vi "test Init 1.vi"(11 "Test Case In":refnum<class "test Init.lvclass">) -> (0 "error out":errorcluster, 3 "Test Case Out":refnum<class "test Init.lvclass">)   [LabVIEW 2023, in "test Init.lvclass"]
uses:
  test Init.lvclass
  test Init.lvclass/test Init.ctl
  <vilib>/Astemes/LUnit/Test Case.lvclass
  source/Base Graph/Base Graph.lvclass
panel:
  out "Intensity Graph":dbl[][](graph)
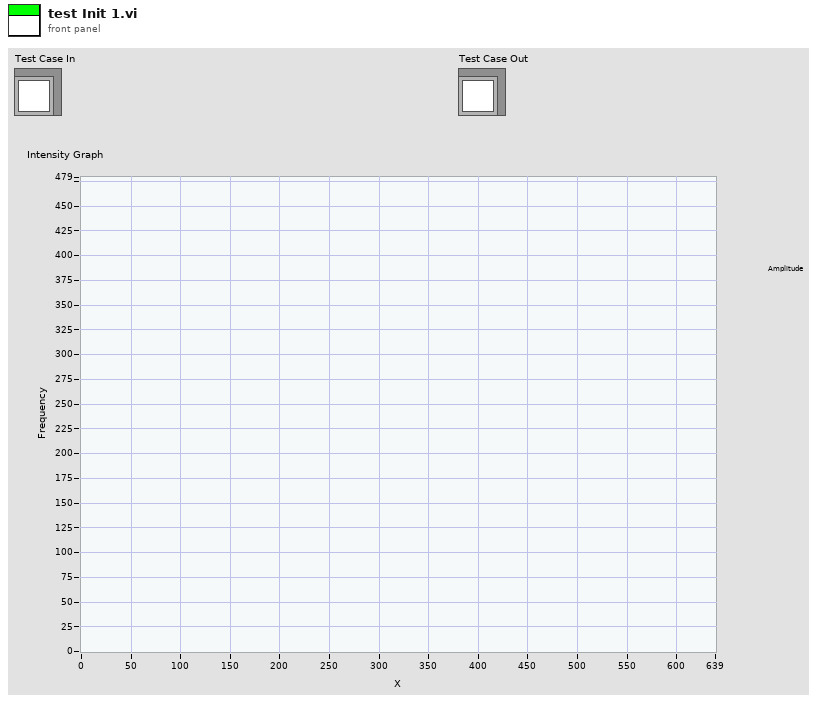
[diagram p1: front panel]
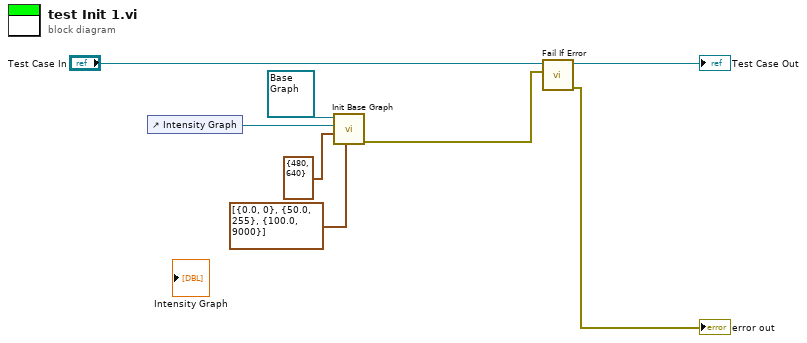
[diagram p0: block diagram]
diagram:
  n1 = control-ref of="Intensity Graph"() -> (w5:refnum<vi>)
  n2 = call "Init Base Graph.vi"("Z Scale.Marker Values[]"=cluster{"Numeric":dbl, "Numeric":u32}[] [{"Numeric"=0.0, "Numeric"=0}, {"Numeric"=50.0, "Numeric"=255}, {"Numeric"=100.0, "Numeric"=9000}], "Size"=cluster{"Height":u32, "Width":u32} {"Height"=480, "Width"=640}, "Intensity Graph"=w5, "Base Graph in"=refnum<class "Base Graph.lvclass"> refnum ("TG Base Graph in")) -> ("error out"=w1:errorcluster)  [unwired: 6 in, 1 out]
  n3 = call <vilib>:"Fail If Error.vi"("Assert error"=w1, "LUnit Test Case In"="Test Case In") -> ("error out"=→"error out":errorcluster, "LUnit Test Case Out"=→"Test Case Out":refnum<class "test Init.lvclass">)  [unwired: 8 in]
